vi "CalculateRoiMetrics.vi"(8 "error in (no error)":errorcluster, 10 "rois":T6[](array[typedef]), 11 "data":T2) -> (0 "error out":errorcluster, 1 "roi cache":variant, 3 "data out":T2, 5 "image status":string)   [LabVIEW 2017, in "IrAnalysis.lvlib"]
uses:
  <vilib>/addons/InsightCM/Devices/Shared/Ir/IrAnalysis/IrAnalysis.lvlib
  <vilib>/addons/InsightCM/Devices/Shared/Ir/IrAnalysis/controls/roi.ctl
  <vilib>/addons/InsightCM/Devices/Shared/Ir/IrAnalysis/controls/metric.ctl
  <vilib>/addons/InsightCM/MessageBus/Base/controls/MetricDefinitionInstance.ctl
  <vilib>/addons/InsightCM/MessageBus/Base/controls/KeyValuePair.ctl
  <vilib>/addons/InsightCM/Devices/Shared/Common/DataFlow/controls/Data.ctl
  <vilib>/addons/InsightCM/Utilities/DataAccessors/controls/wfmSGL_DVR.ctl
  <vilib>/addons/PointValueMap/controls/PointMap.ctl
  <vilib>/addons/InsightCM/Devices/Shared/Common/DataFlow/controls/Type.ctl
  <vilib>/addons/PointValueMap/subVIs/Point_Write_double.vi
  <vilib>/addons/InsightCM/Utilities/PropertyHelpers/PropertyHelpers.lvlib
  <vilib>/vision/NI_Vision_Development_Module.lvlib
  <vilib>/addons/PointValueMap/PointValueMap.lvlib
  <vilib>/addons/InsightCM/Devices/Shared/Common/DataFlow/DataFlow.lvlib
panel:
  out "image":T1(plugin-control)
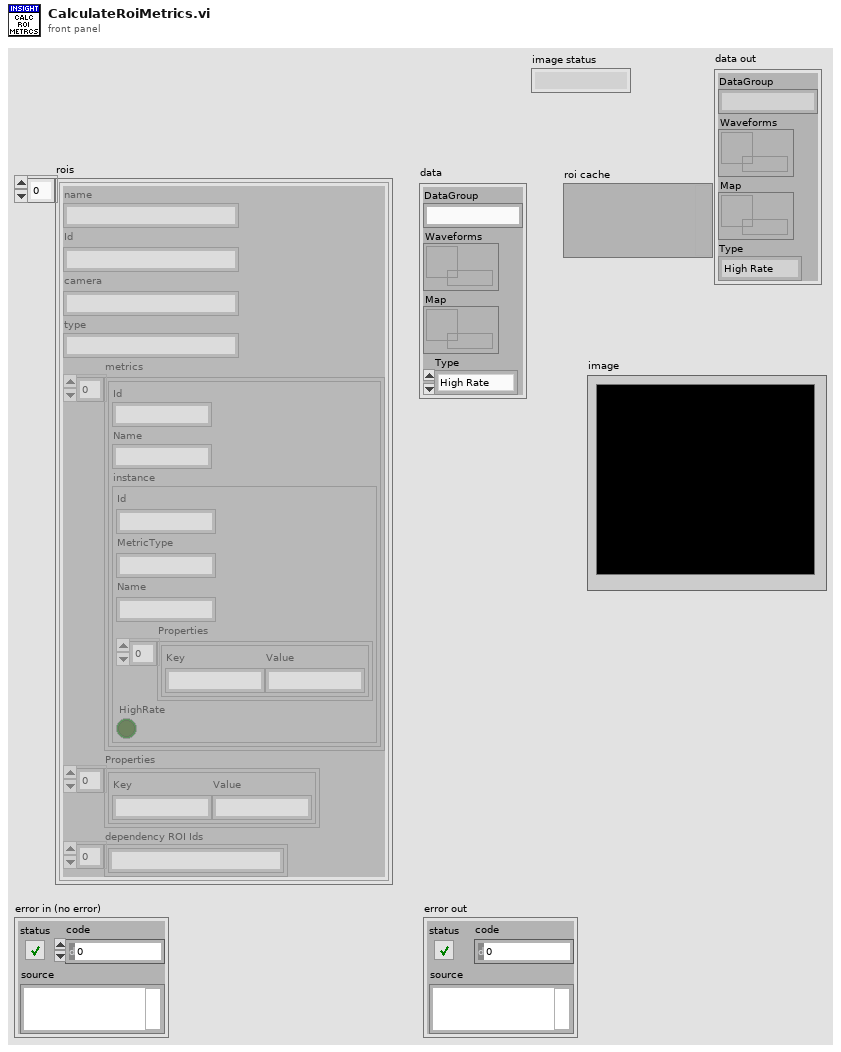
[diagram p1: front panel]
types:
  T1 = typedef "IMAQ Image.ctl" = refnum<image>
  T2 = typedef "DataFlow.lvlib/Data.ctl" = cluster{"DataGroup":string, "Waveforms":T3, "Map":T4, "Type":T5}
  T3 = typedef "wfmSGL_DVR.ctl" = refnum<data-value>
  T4 = typedef "PointValueMap.lvlib/PointMap.ctl" = refnum<data-value>
  T5 = typedef "DataFlow.lvlib/Type.ctl" = enum16{"High Rate", "Low Rate", "Burst Mode"}
  T6 = typedef "IrAnalysis.lvlib/roi.ctl" = cluster{"name":string, "Id":string, "camera":string, "type":string, "metrics":T7[], "Properties":T9[], "dependency ROI Ids":string[]}
  T7 = typedef "IrAnalysis.lvlib/metric.ctl" = cluster{"Id":string, "Name":string, "instance":T8}
  T8 = typedef "MetricDefinitionInstance.ctl" = cluster{"Id":string, "MetricType":string, "Name":string, "Properties":T9[], "HighRate":bool}
  T9 = typedef "KeyValuePair.ctl" = cluster{"Key":string, "Value":string}
  T10 = cluster{"Global Rectangle":i32[], "Contours":cluster{"Contour Type":u32, "ROI Type":u32, "Points":i32[]}[]}
  T11 = typedef "Image Type" = u32
  T12 = cluster{"Mean Value":sgl, "Standard Variation":sgl, "Minimal Value":sgl, "Maximal Value":sgl, "Area (calibrated)":sgl, "Area (pixels)":u32, "%":sgl, "Calibration Valid":bool}
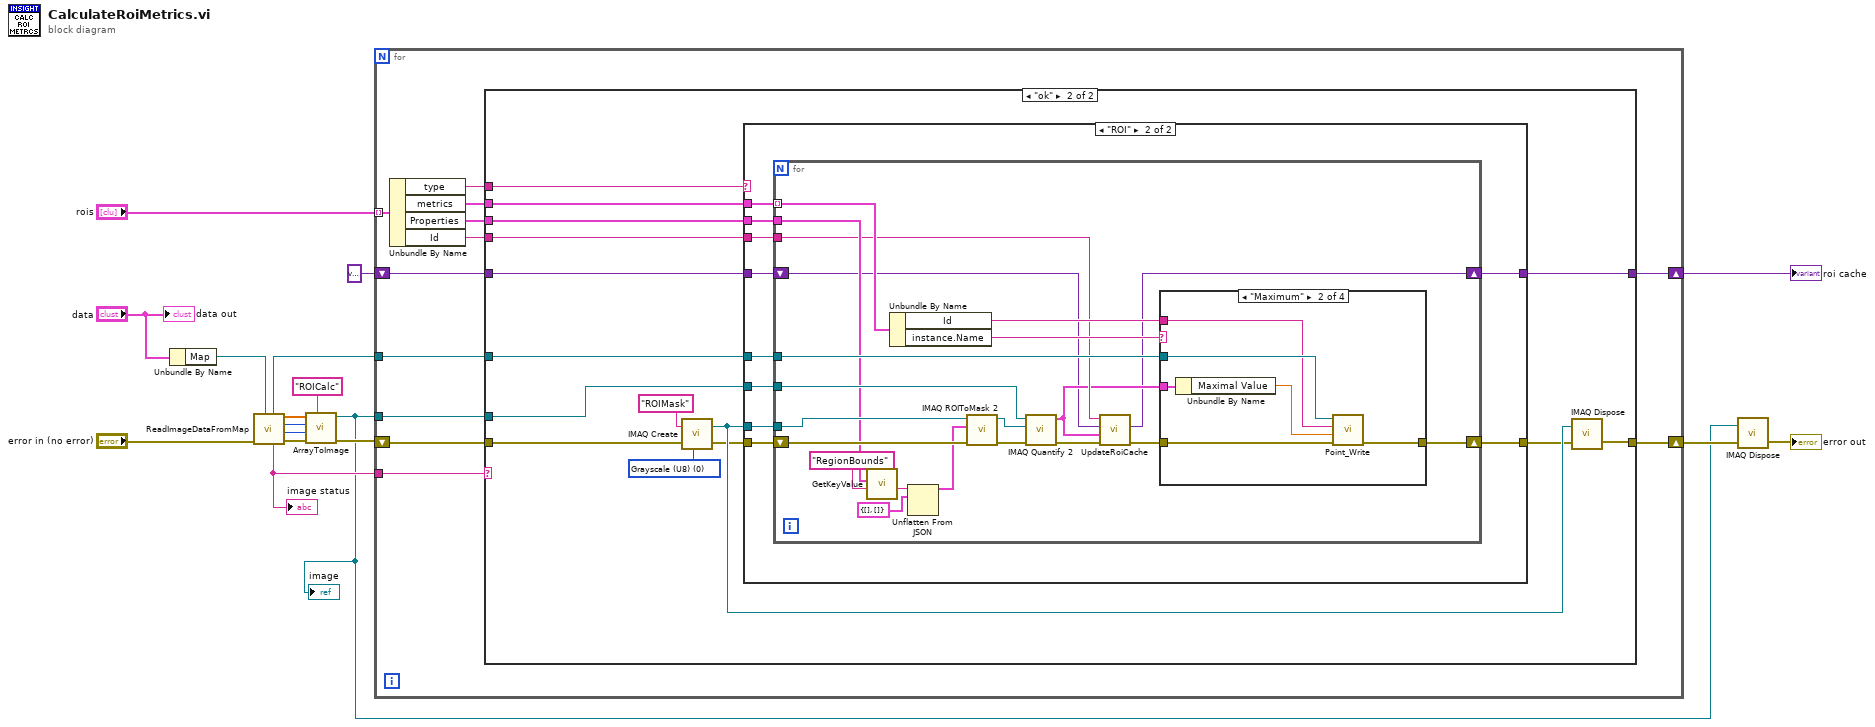
[diagram p0: block diagram]
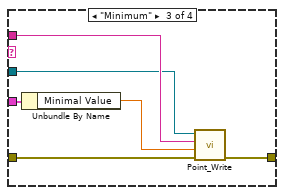
[diagram p5: hidden frame]
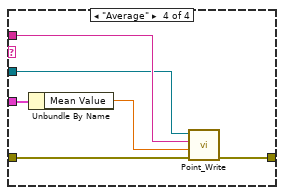
[diagram p6: hidden frame]
diagram:
  n1 = Unbundle By Name("data") -> ("Map"=w7:T4)
  n2 = call <vilib>:"ReadImageDataFromMap.vi"("map"=w7, "error in (no error)"="error in (no error)") -> ("error out"=w8:errorcluster, "image height"=w9:i32, "image width"=w10:i32, "image data"=w11:sgl[], "image status"=w12:string, "map out"=w5:T4)  [unwired: 3 in, 1 out]
  "image status" <- w12
  n3 = call <vilib>:"ArrayToImage.vi"("image name"="ROICalc", "error in (no error)"=w8, "height"=w9, "width"=w10, "image data"=w11) -> ("error out"=w6:errorcluster, "image"=w1:T1)  [unwired: 5 in]
  "image" <- w1
  n4 = for {
    shift-right: [w29] -> w3
    shift-left: w6 -> [w21]
    tunnel: "rois" -> [w25] mode=indexing
    shift-right: [w22] -> w16
    shift-left: variant -> [w23]
    tunnel: w12 -> [w19]
    tunnel: w1 -> [w20]
    tunnel: w5 -> [w18]
    n5 = Unbundle By Name(w25) -> ("type"=w27:string, "metrics"=w28:T7[], "Properties"=w26:T9[], "Id"=w24:string)
    n6 = case shown="\"ok\"" w19 {
      tunnel: w28 -> [_ w43]
      tunnel: [w31 w32] -> w29
      tunnel: w21 -> [w31 w34]
      tunnel: w27 -> [_ w42]
      tunnel: w26 -> [_ w39]
      tunnel: w24 -> [_ w38]
      tunnel: w23 -> [w30 w37]
      tunnel: [w30 w36] -> w22
      tunnel: w20 -> [_ w33]
      tunnel: w18 -> [_ w35]
      frame "", Default {
      }
      frame "ok" {
        w46 = T11 0 items=["Grayscale (U8)", "Grayscale (I16)", "Grayscale (SGL)", "Complex (CSG)", "RGB (U32)", "HSL (U32)", "RGB (U64)", "Grayscale (U16)"] ("Image Type")
        n7 = call "IMAQ Create"("Image Name"="ROIMask", "Image Type"=w46, "error in (no error)"=w34) -> ("New Image"=w44:T1, "error out"=w41:errorcluster)  [unwired: 2 in]
        n8 = case shown="\"ROI\"" w42 {
          tunnel: w43 -> [_ w58]
          tunnel: w35 -> [_ w57]
          tunnel: w41 -> [w48 w56]
          tunnel: w33 -> [_ w54]
          tunnel: [w48 w53] -> w40
          tunnel: w44 -> [_ w55]
          tunnel: w39 -> [_ w52]
          tunnel: w38 -> [_ w51]
          tunnel: w37 -> [w47 w50]
          tunnel: [w47 w49] -> w36
          frame "", Default {
          }
          frame "ROI" {
            n9 = for {
              tunnel: w58 -> [w79] mode=indexing
              tunnel: w57 -> [w78]
              tunnel: w55 -> [w72]
              tunnel: w54 -> [w71]
              tunnel: w52 -> [w67]
              tunnel: w51 -> [w64]
              shift-right: [w68] -> w53
              shift-left: w56 -> [w73]
              shift-right: [w61] -> w49
              shift-left: w50 -> [w62]
              n10 = call <vilib>:"GetKeyValue.vi"("key"="RegionBounds", "key value pairs"=w67) -> ("value"=w77:string)  [unwired: 7 in, 2 out]
              n11 = Unbundle By Name(w79) -> ("Id"=w69:string, "instance.Name"=w70:string)
              n12 = Unflatten From JSON(JSON string=w77, type and defaults=T10 {"Global Rectangle"=[], "Contours"=[]} ("bounds")) -> (value=w60:T10)  [unwired: 5 in, 1 out]
              n13 = call "IMAQ ROIToMask 2"("error in (no error)"=w73, "ROI Descriptor"=w60, "Image"=w72) -> ("error out"=w75:errorcluster, "Image Out"=w74:T1)  [unwired: 6 in, 1 out]
              n14 = call "IMAQ Quantify 2"("error in (no error)"=w75, "Image Mask"=w74, "Image"=w71) -> ("error out"=w65:errorcluster, "Global Report"=w63:T12)  [unwired: 6 in, 1 out]
              n15 = call <vilib>:"UpdateRoiCache.vi"("error in (no error)"=w65, "Global Report"=w63, "roi cache in"=w62, "roi id"=w64) -> ("error out"=w66:errorcluster, "roi cache out"=w61:variant)  [unwired: 6 in]
              n16 = case shown="\"Maximum\"" w70 {
                tunnel: w69 -> [_ w83 w92 w97]
                tunnel: w78 -> [_ w85 w87 w93]
                tunnel: w63 -> [_ w81 w91 w96]
                tunnel: w66 -> [w80 w86 w89 w95]
                tunnel: [w80 w82 w88 w94] -> w68
                frame "", Default {
                }
                frame "Maximum" {
                  n17 = Unbundle By Name(w81) -> ("Maximal Value"=w84:sgl)
                  n18 = call-poly <vilib>:"Point_Write.vi"("Error In"=w86, "Value"=w84, "Tag"=w83, "Map"=w85) -> ("Error Out"=w82:errorcluster)  [unwired: 6 in, 1 out]
                }
                frame "Minimum" {
                  n19 = Unbundle By Name(w91) -> ("Minimal Value"=w90:sgl)
                  n20 = call-poly <vilib>:"Point_Write.vi"("Error In"=w89, "Value"=w90, "Tag"=w92, "Map"=w87) -> ("Error Out"=w88:errorcluster)  [unwired: 6 in, 1 out]
                }
                frame "Average" {
                  n21 = Unbundle By Name(w96) -> ("Mean Value"=w98:sgl)
                  n22 = call-poly <vilib>:"Point_Write.vi"("Error In"=w95, "Value"=w98, "Tag"=w97, "Map"=w93) -> ("Error Out"=w94:errorcluster)  [unwired: 6 in, 1 out]
                }
              }
            }
          }
        }
        n23 = call "IMAQ Dispose"("Image"=w44, "error in (no error)"=w40) -> ("error out"=w32:errorcluster)  [unwired: 4 in]
      }
    }
  }
  "roi cache" <- w16
  n24 = call "IMAQ Dispose"("Image"=w1, "error in (no error)"=w3) -> ("error out"=→"error out":errorcluster)  [unwired: 4 in]
  "data out" <- "data"
